vi "S8300E_USB_IF_TEST_WIH.vi"() -> ()   [LabVIEW 2011]
panel:
  out "LOG2":string
  out "LOG1":string
  out "CMD-LIST":cluster{string, string, string, string}[](array[cluster])
  out "log msg":string
  out "VISA resource name out":refnum<visa-resource-name>
  out "BEGIN TIME":u32
  out "進行狀況":string
  # "Error Code:USB-IF2\nError Code:USB-IF3"
  # "2015-6-2"
  # "S8300E USB Interface Test(接UART COM9)"
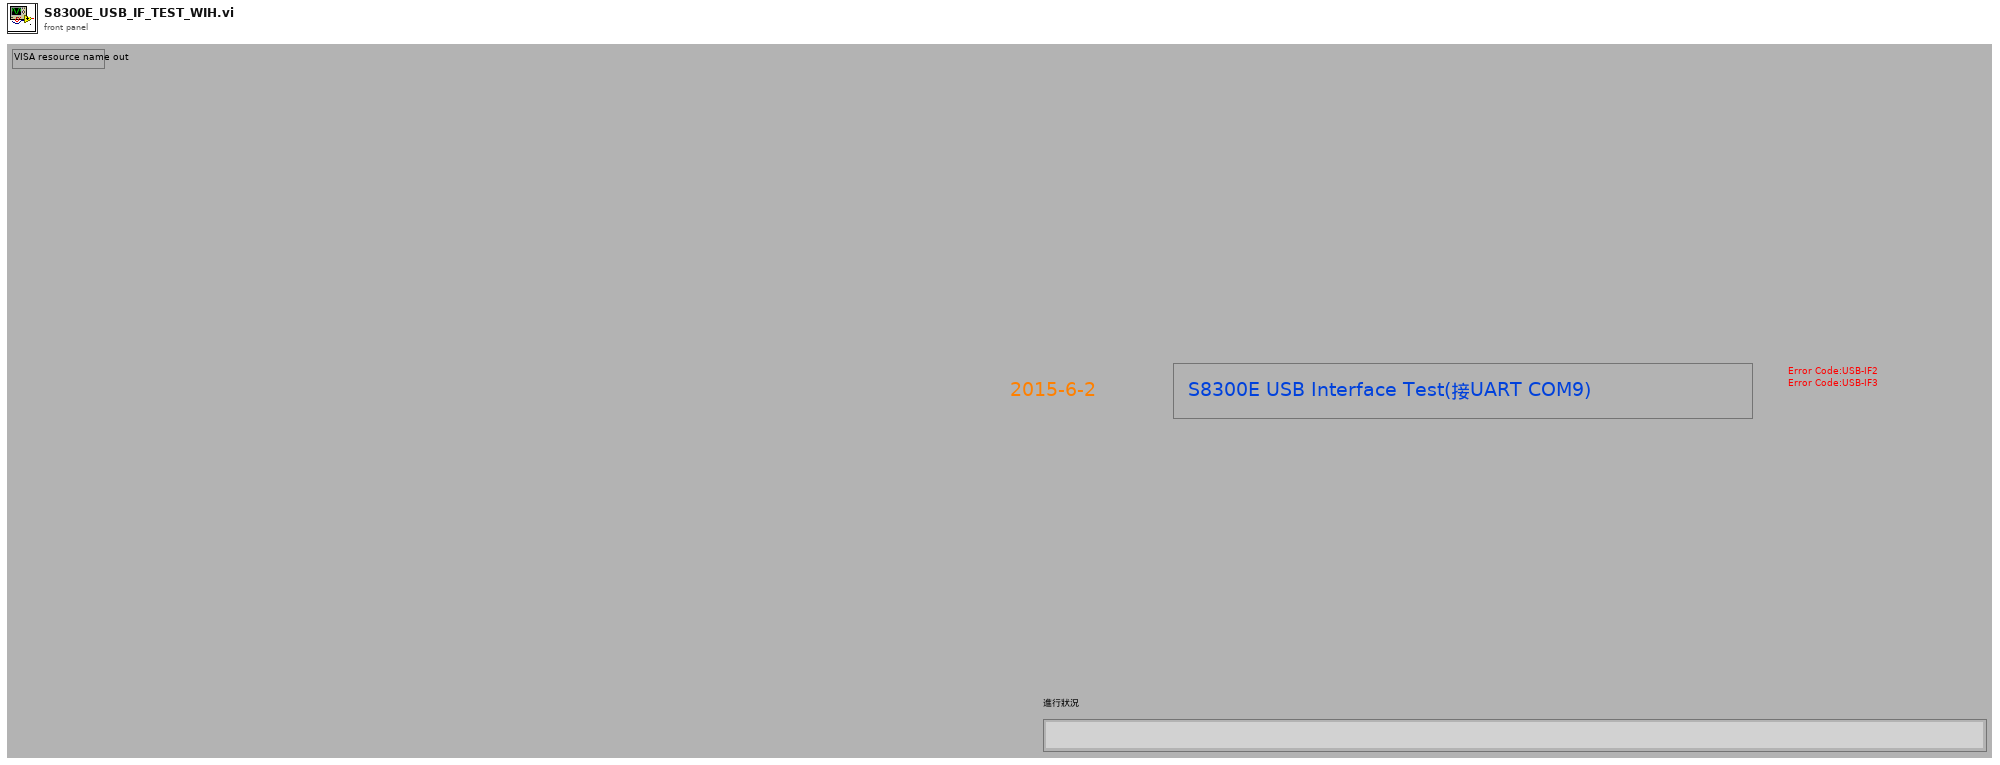
[diagram p1: front panel]
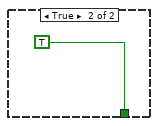
[diagram p7: hidden frame]
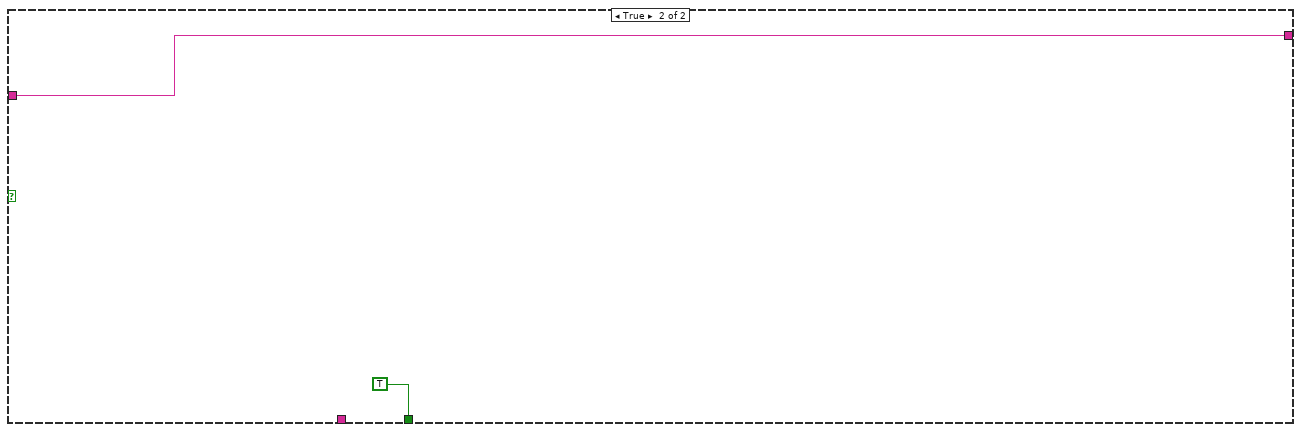
[diagram p9: hidden frame]
diagram:
  n1 = flat-sequence {
    frame #0 {
      n2 = Tick Count (ms)() -> (millisecond timer value=→"BEGIN TIME":u32)
    }
    frame #1 {
      n3 = property on="進行狀況" class="Str"("Blinking"=TRUE) -> ()  [unwired: 2 in, 2 out]
      "進行狀況" <- "進入測試準備中...." ("進行狀況")
    }
    frame #2 {
      n4 = call "SUB_SearchFile_inFolder.vi"("Search Filename in Folder"="S8300E_sfcs_misc.txt") -> ("File Existing True/Flase"=w4:bool)  [unwired: 1 in]
      n5 = case shown="False" w4 {
        frame False {
          n6 = flat-sequence {
            frame #0 {
              n7 = call "Display Message to User"() -> ()  [unwired: 10 in, 2 out]
            }
            frame #1 {
              n8 = call "SUB_Writelog.vi"("Pass/Fail"="Fail:S8300E_USB_IF_TEST") -> ()  [unwired: 2 in]
            }
            frame #2 {
              n9 = Quit LabVIEW(quit? (T)=TRUE) -> ()
            }
          }
        }
        frame True {
        }
      }
    }
    frame #3 {
      n10 = Concatenate Strings("./usb.sh -t  1", "\r") -> (w26:string)
      n11 = Concatenate Strings("./usb.sh -t  2", "\r") -> (w21:string)
      n12 = Concatenate Strings("./usb.sh -t  3", "\r") -> (w16:string)
      n13 = Bundle(w26, "PASSED=", "Checking USB IF-1...", "USB-IF1") -> ()  [unwired: 1 in, 1 out]
      n14 = Bundle(w21, "PASSED=", "Checking USB IF-2...", "USB-IF2") -> (w10:cluster{string, string, string, string})  [unwired: 1 in]
      n15 = Bundle(w16, "PASSED=", "Checking USB IF-3...", "USB-IF3") -> (w9:cluster{string, string, string, string})  [unwired: 1 in]
      n16 = Build Array(w10, w9) -> (→"CMD-LIST":cluster{string, string, string, string}[])
    }
    frame #4 {
      n17 = case shown="True" TRUE {
        frame False {
        }
        frame True {
          n18 = call "SUB_COM1_CLOSE.vi"("VISA resource name"=refnum<visa-resource-name> "COM9") -> ()  [unwired: 3 in]
        }
      }
    }
    frame #5 {
      n19 = case shown="True" TRUE {
        frame False {
        }
        frame True {
          n20 = call "SUB_COM9_INIT.vi"("baud rate"=u32 115200) -> ("VISA resource name out"=w35:refnum<visa-resource-name>)  [unwired: 1 in, 1 out]
          "VISA resource name out" <- w35
          n21 = call "SUB_COM1Wrt.vi"("VISA resource name"=w35, "write buffer"="\r") -> ("duplicate VISA resource name"=w32:refnum<visa-resource-name>)  [unwired: 1 in, 1 out]
          n22 = call "SUB_ContinueCom1Read.vi"("Numeric"=1200, "duplicate VISA resource name 2"=w32) -> ()  [unwired: 1 in, 3 out]
        }
      }
    }
    frame #6 {
      n23 = case shown="True" TRUE {
        frame False {
        }
        frame True {
          n24 = while {
            shift-right: [w41] -> _
            shift-left: "" -> [w39]
            stop <- w48 stop-if-true
            n25 = local read "VISA resource name out"() -> (w42:refnum<visa-resource-name>)
            n26 = call "SUB_COM1Wrt.vi"("VISA resource name"=w42, "write buffer"="\r") -> ("duplicate VISA resource name"=w47:refnum<visa-resource-name>)  [unwired: 1 in, 1 out]
            n27 = Tick Count (ms)() -> (millisecond timer value=w46:u32)
            n28 = call "SUB_READ_COM1_FindString_timeout.vi"("Find this String"="s8300e_func_test#", "Timeout Seccond"=5.0, "Begin time"=w46, "duplicate VISA resource name 2"=w47) -> ("Output String"=w40:string, "Found String"=w43:bool)  [unwired: 1 in, 1 out]
            n29 = case shown="False" w43 {
              tunnel: [w53 TRUE] -> w48
              tunnel: w40 -> [w51 _]
              frame False {
                w52 = "UART無正確反應!需有S8300E字串" ("Status")
                n30 = call "SUB_YESNO.vi"("Debug View"=w51, "Status"=w52) -> ("yes/no"=w56:enum32{"No Selection", "Yes", "No", "None"})  [unwired: 1 in]
                n31 = Concatenate Strings(w52, w51) -> (w50:string)
                n32 = Equal?(x=w56, y=enum32{"No Selection", "Yes", "No", "None"}."No") -> (x = y?=w54:bool)
                n33 = case shown="True" w54 {
                  tunnel: [_ w58] -> w53
                  tunnel: w50 -> [_ w57]
                  frame False {
                  }
                  frame True {
                    n34 = flat-sequence {
                      tunnel: w57 -> [w61]
                      tunnel: [w66] -> w58
                      frame #0 {
                        n35 = local read "LOG1"() -> (w59:string)
                        n36 = Concatenate Strings("Fail:S8300E_USB_IF_TEST" ("Pass/Fail"), "\n", w61, w59) -> (w60:string)
                        n37 = call "SUB_Writelog.vi"("Pass/Fail"=w60) -> ()  [unwired: 2 in]
                      }
                      frame #1 {
                        n38 = call "SUB_SFCS_SendResult.vi"("ErrorCode"="UART", "PASS_Fail (1/0)"=i8 0) -> ()  [unwired: 1 out]
                      }
                      frame #2 {
                        w66 = TRUE ("quit? (T)")
                        n39 = Quit LabVIEW(quit? (T)=w66) -> ()
                      }
                    }
                  }
                }
              }
              frame True {
              }
            }
            n40 = Concatenate Strings(w39, w40) -> (w41:string)
            "LOG1" <- w41
          }
        }
      }
    }
    frame #7 {
      n41 = local read "CMD-LIST"() -> (w68:cluster{string, string, string, string}[])
      n42 = Array Size(array=w68) -> (size(s)=w71:i32)
      n43 = for {
        N: w71 -> [_]
        shift-right: [w73] -> w69
        shift-left: "" -> [w72]
        i -> [w76]
        n44 = while {
          tunnel: w76 -> [w97]
          shift-right: [w82] -> w74
          shift-left: "" -> [w80]
          stop <- w92 stop-if-true
          n45 = local read "CMD-LIST"() -> (w91:cluster{string, string, string, string}[])
          n46 = local read "VISA resource name out"() -> (w78:refnum<visa-resource-name>)
          n47 = Index Array(array=w91, index=w97) -> (element=w90:cluster{string, string, string, string})
          n48 = call "SUB_ContinueCom1Read.vi"("Numeric"=2400, "duplicate VISA resource name 2"=w78) -> ("duplicate VISA resource name"=w77:refnum<visa-resource-name>)  [unwired: 1 in, 2 out]
          n49 = Unbundle(w90) -> (w86:string, w88:string, w89:string, w87:string)
          n50 = call "SUB_COM1Wrt.vi"("VISA resource name"=w77, "write buffer"=w86) -> ("duplicate VISA resource name"=w96:refnum<visa-resource-name>)  [unwired: 1 in, 1 out]
          n51 = Tick Count (ms)() -> (millisecond timer value=w95:u32)
          n52 = call "SUB_READ_COM1_FindString_timeout.vi"("Find this String"=w88, "Timeout Seccond"=8.0, "Begin time"=w95, "duplicate VISA resource name 2"=w96) -> ("Output String"=w84:string, "Found String"=w93:bool)  [unwired: 1 in, 1 out]
          n53 = Concatenate Strings(w86, "\n", w84) -> (w83:string)
          n54 = local write "進行狀況"(w89) -> ()
          n55 = case shown="False" w93 {
            tunnel: [_ TRUE] -> w92
            tunnel: w87 -> [w105 _]
            tunnel: [w99 w124] -> w81
            tunnel: w83 -> [w100 w124]
            frame False {
              n56 = local read "進行狀況"() -> (w102:string)
              n57 = Concatenate Strings("USB測試失敗!有接U盤?" ("string"), "\r", w102) -> (w101:string)
              n58 = call "SUB_YESNO.vi"("Debug View"=w100, "Status"=w101) -> ("yes/no"=w108:enum32{"No Selection", "Yes", "No", "None"})  [unwired: 1 in]
              n59 = Equal?(x=w108, y=enum32{"No Selection", "Yes", "No", "None"}."No") -> (x = y?=w106:bool)
              n60 = Concatenate Strings(w101, w100) -> (w98:string)
              n61 = case shown="True" w106 {
                tunnel: w105 -> [_ w112]
                tunnel: w98 -> [_ w111]
                tunnel: [w109 w110] -> w99
                tunnel: w98 -> [w109 w110]
                frame False {
                }
                frame True {
                  n62 = flat-sequence {
                    tunnel: [w119] -> w113
                    tunnel: w112 -> [w119]
                    tunnel: w111 -> [w117]
                    tunnel: w113 -> [w120]
                    frame #0 {
                      w116 = "\n"
                      n63 = local read "LOG2"() -> (w115:string)
                      n64 = Concatenate Strings("Fail:S8300E_USB_IF_TEST" ("Pass/Fail"), w116, w117, w116, w115) -> (w114:string)
                      n65 = call "SUB_Writelog.vi"("Pass/Fail"=w114) -> ()  [unwired: 2 in]
                    }
                    frame #1 {
                      n66 = call "SUB_SFCS_SendResult.vi"("ErrorCode"=w120, "PASS_Fail (1/0)"=i8 0) -> ()  [unwired: 1 out]
                    }
                    frame #2 {
                      n67 = call "SUB_COM1_CLOSE.vi"("VISA resource name"=refnum<visa-resource-name> "COM9") -> ()  [unwired: 3 in]
                    }
                    frame #3 {
                      n68 = Quit LabVIEW(quit? (T)=TRUE) -> ()
                    }
                  }
                }
              }
            }
            frame True {
            }
          }
          n69 = Concatenate Strings(w80, w81) -> (w82:string)
          "LOG2" <- w82
        }
        n70 = Concatenate Strings(w72, w74) -> (w73:string)
      }
      "log msg" <- w69
    }
    frame #8 {
      n71 = call "SUB_COM1_CLOSE.vi"("VISA resource name"=refnum<visa-resource-name> "COM9") -> ()  [unwired: 3 in]
    }
    frame #9 {
      w129 = "***Not Good ***" ("replace string (\"\")")
      n72 = local read "log msg"() -> (w133:string)
      n73 = local read "BEGIN TIME"() -> (w138:u32)
      n74 = Tick Count (ms)() -> (millisecond timer value=w137:u32)
      n75 = call "SUB_CAL_TESTTIME.vi"("Test Item name"="S8300E_USB_IF_TEST", "Stop tick time"=w137, "Start tick time"=w138) -> ("Test Time output"=w135:string)  [unwired: 2 in]
      n76 = Concatenate Strings("Pass:S8300E_USB_IF_TEST", "\n", w133, w135) -> (w128:string)
      n77 = call "SUB_SEARCH_REPLACE_STR.vi"("replace string (\"\")"=w129, "search string"="FAILED", "input string"=w128) -> ("result string"=w131:string)  [unwired: 2 in]
      n78 = call "SUB_SEARCH_REPLACE_STR.vi"("replace string (\"\")"=w129, "search string"="FAIL", "input string"=w131) -> ("result string"=w127:string)  [unwired: 2 in]
      n79 = call "SUB_Writelog.vi"("Pass/Fail"=w127) -> ()  [unwired: 2 in]
    }
    frame #10 {
      n80 = Quit LabVIEW(quit? (T)=TRUE ("stop? (T)")) -> ()
    }
  }
